vi "VF_DeviceID Zero Fault.vi"(7 "VF DeviceID 0?":bool, 11 "IED_Status_ID in":T1) -> (3 "IED_Status_ID out":T1)   [LabVIEW 2018]
uses:
  <vilib>/ORNL/CSEISMIC DDS/CSEISMIC DDS Base/Data Types/IED_Status.ctl
  <vilib>/ORNL/CSEISMIC DDS/CSEISMIC DDS Base/Data Types/Controls/DeviceID.ctl
  <vilib>/ORNL/CSEISMIC DDS/CSEISMIC DDS Base/Data Types/Controls/Timestamp.ctl
  <vilib>/ORNL/CSEISMIC DDS/CSEISMIC DDS Base/CSEISMIC DDS.lvclass
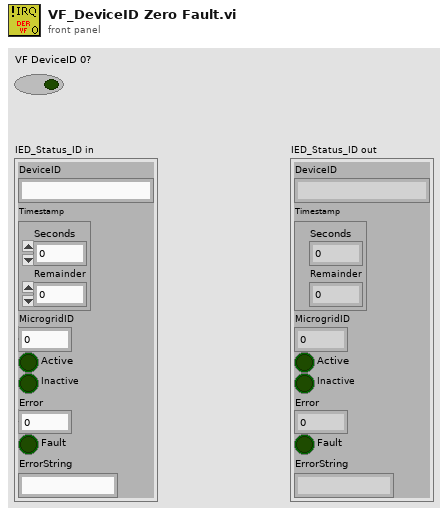
[diagram p1: front panel]
types:
  T1 = typedef "CSEISMIC DDS.lvlib/CSEISMIC DDS.lvclass/IED_Status.ctl" = cluster{"DeviceID":T2, "Timestamp":T3, "MicrogridID":u8, "Active":bool, "Inactive":bool, "Error":i32, "Fault":bool, "ErrorString":string}
  T2 = typedef "CSEISMIC DDS.lvlib/CSEISMIC DDS.lvclass/DeviceID.ctl" = string
  T3 = typedef "CSEISMIC DDS.lvlib/CSEISMIC DDS.lvclass/Timestamp.ctl" = cluster{"Seconds":u64, "Remainder":u64}
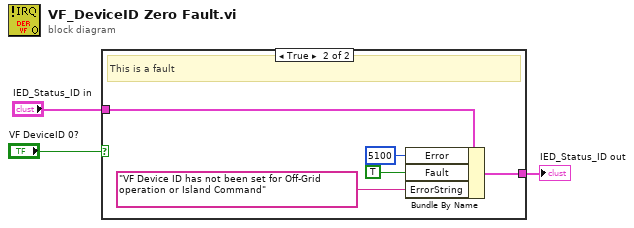
[diagram p0: block diagram]
diagram:
  n1 = case shown="True" "VF DeviceID 0?" {
    tunnel: [w4 w6] -> w2
    tunnel: "IED_Status_ID in" -> [w4 w5]
    frame False {
      # "This is expected"
    }
    frame True {
      # "This is a fault"
      n2 = Bundle By Name(cluster=w5, "Error"=5100, "Fault"=TRUE, "ErrorString"="VF Device ID has not been set for Off-Grid operation or Island Command") -> (w6:T1)
    }
  }
  "IED_Status_ID out" <- w2
